vi "Do.vi"(8 "error in":errorcluster, 10 "Actor in":refnum<class "Actor.lvclass">, 11 "Initialize Alicat SP MSG":refnum<class "Initialize Device SP MSG.lvclass">) -> (0 "error out":errorcluster, 2 "Actor out":refnum<class "Actor.lvclass">)   [LabVIEW 2016, in "Controller.lvlib" / "Initialize Device SP MSG.lvclass"]
doc: "(<B>Filename</B>: Actor Framework.lvlib:Message.lvclass:Do.vi)\n\nDefines what a message does when it is received by an actor. Generally, a message instructs an actor to invoke one of its methods. By default, this method does nothing. A child class must override it to define behavior. Create a child class by using the Actor Framework Message Maker dialog box."
uses:
  Initialize Device SP MSG.lvclass
  C:/Program Files (x86)/National Instruments/LabVIEW 2016/vi.lib/MSR Consulting, LLC/Devices/DAQ Device/Messages/Generic CVT Init/Generic Init CVT Message.lvclass
  <vilib>/ActorFramework/Actor/Actor.lvclass
  <vilib>/MSR Consulting, LLC/General Reuse/SuperActor/SuperActor.lvclass
  C:/Program Files (x86)/National Instruments/LabVIEW 2016/vi.lib/ActorFramework/Actor/Actor.lvclass
  <vilib>/MSR Consulting, LLC/General Reuse/SuperActor/SuperActor.lvclass/SuperActor.ctl
  <vilib>/MSR Consulting, LLC/Devices/DAQ Device/Messages/Generic CVT Init/Generic Init CVT Message.lvclass/Generic Init CVT Message.ctl
  <vilib>/MSR Consulting, LLC/General Reuse/SuperActor/Read CVT Session.vi
  <vilib>/MSR Consulting, LLC/General Reuse/SuperActor/Read Log Session.vi
  <vilib>/MSR Consulting, LLC/Devices/DAQ Device/Messages/Generic CVT Init/Read DevID.vi
  <vilib>/MSR Consulting, LLC/Devices/DAQ Device/Messages/Generic CVT Init/Read SP.vi
  <vilib>/MSR Consulting, LLC/General Reuse/Session APIs/_Session Fwk/Session - Root.lvclass
  <vilib>/MSR Consulting, LLC/General Reuse/Session APIs/CVT/CVT.lvclass
  <vilib>/MSR Consulting, LLC/General Reuse/Session APIs/Session Log/System Log.lvclass
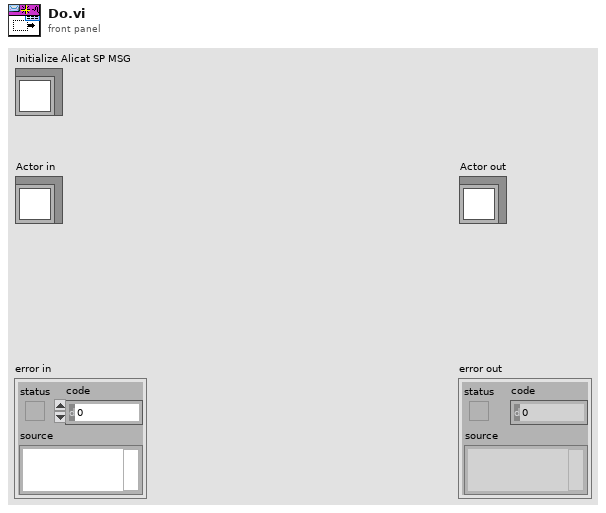
[diagram p1: front panel]
types:
  T1 = typedef "Session - Root.lvclass/Session Handle.ctl" = refnum<data-value>
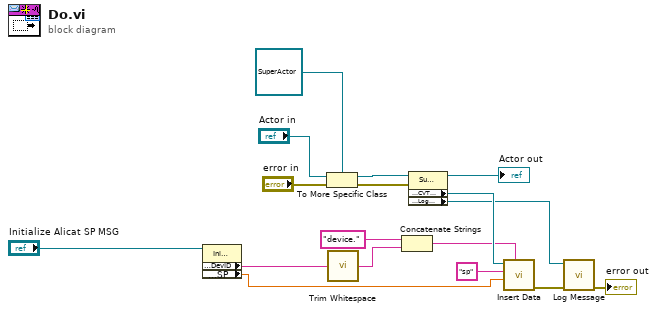
[diagram p0: block diagram]
diagram:
  n1 = property class="Initialize Alicat SP MSG"(reference="Initialize Alicat SP MSG") -> ("Accessors:DevID"=w5:string, "Accessors:SP"=w9:dbl)  [unwired: 1 in, 2 out]
  n2 = To More Specific Class(target class=refnum<class "SuperActor.lvclass"> refnum ("SuperActor.lvlib:SuperActor"), reference="Actor in", error in="error in") -> (specific class reference=w15:refnum<class "SuperActor.lvclass">, error out=w14:errorcluster)
  n3 = call <vilib>:"Trim Whitespace.vi"("string"=w5) -> ("trimmed string"=w4:string)  [unwired: 1 in]
  n4 = Concatenate Strings("device." ("Group"), w4) -> (w7:string)
  n5 = property class="SuperActor"(reference=w15, error in=w14) -> (reference out=→"Actor out":refnum<class "SuperActor.lvclass">, "Accessors:CVT Session"=w10:T1, "Accessors:Log Session"=w3:T1)  [unwired: 1 out]
  n6 = call <vilib>:"Insert Data.vi"("Group"=w7, "Data"=w9, "tag"="sp", "CVT Session In"=w10) -> ("error out"=w2:errorcluster)  [unwired: 6 in, 1 out]
  n7 = call <vilib>:"Log Message.vi"("error in"=w2, "session in"=w3) -> ("error out"=→"error out":errorcluster)  [unwired: 8 in, 1 out]
